vi "Test - Texture Mapping Test 1.vi"() -> ()   [LabVIEW 2020, in "3D.lvlib"]
uses:
  3D.lvlib
  Utility/Utility.lvlib
  Raster/Raster.lvlib
  Vector 3D.ctl
  Triangle 3D With Colour.ctl
  Raster/Rectangle Dimensions.ctl
  Camera.ctl
panel:
  in  "x Rotation":sgl(slide) scale=-180.0..180.0
  in  "y Rotation":sgl(slide) scale=0.0..360.0
  in  "z Rotation":sgl(slide) scale=-180.0..180.0
  in  "x Transform":sgl(slide) scale=-10.0..10.0
  in  "y Transform":sgl(slide)=5.0 scale=-10.0..10.0
  in  "z Transform":sgl(slide)=-18.0 scale=-20.0..10.0
  out "2D Picture":picture
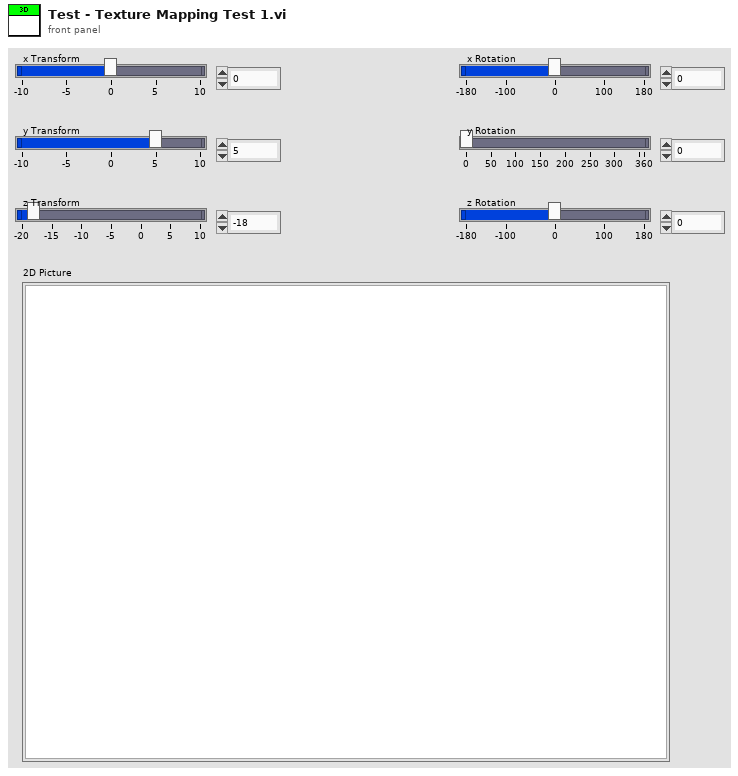
[diagram p1: front panel]
types:
  T1 = typedef "3D.lvlib/Vector 3D.ctl" = cluster{"x":sgl, "y":sgl, "z":sgl}
  T2 = typedef "3D.lvlib/Camera.ctl" = cluster{"Field Of View":sgl, "Near Plane":sgl, "Far Plane":sgl}
  T3 = typedef "Raster.lvlib/Rectangle Dimensions.ctl" = cluster{"Width":u32, "Height":u32}
  T4 = typedef "3D.lvlib/Object.ctl" = cluster{"Triangles":T5[], "Transform":T10, "Name":string, "Alpha Blending Enabled":bool, "Alpha":dbl, "Turntable Enabled":bool, "Material":T8}
  T5 = typedef "3D.lvlib/Triangle.ctl" = cluster{"Vertex 1":T6, "Vertex 2":T6, "Vertex 3":T6, "Alpha":dbl, "Alpha Blending Enabled":bool, "Colour":u32, "Material":T8}
  T6 = typedef "3D.lvlib/Vertex.ctl" = cluster{"Position":T1, "UV":T7, "Colour":u32}
  T7 = typedef "Raster.lvlib/UV.ctl" = cluster{"u":sgl, "v":sgl}
  T8 = typedef "3D.lvlib/Material.ctl" = cluster{"Diffuse Colour":u32, "Texture":T9}
  T9 = typedef "Raster.lvlib/Texture.ctl" = cluster{"Pixels":refnum<data-value>, "Size":T3}
  T10 = typedef "3D.lvlib/Transform.ctl" = cluster{"Position":T1, "Rotation":T1, "Scale":T1}
  T11 = typedef "3D.lvlib/Triangle 3D With Colour.ctl" = cluster{"Point 1":T1, "Point 2":T1, "Point 3":T1, "Fill Colour":u32, "Alpha":dbl, "Alpha Blending Enabled":bool, "Index":i32}
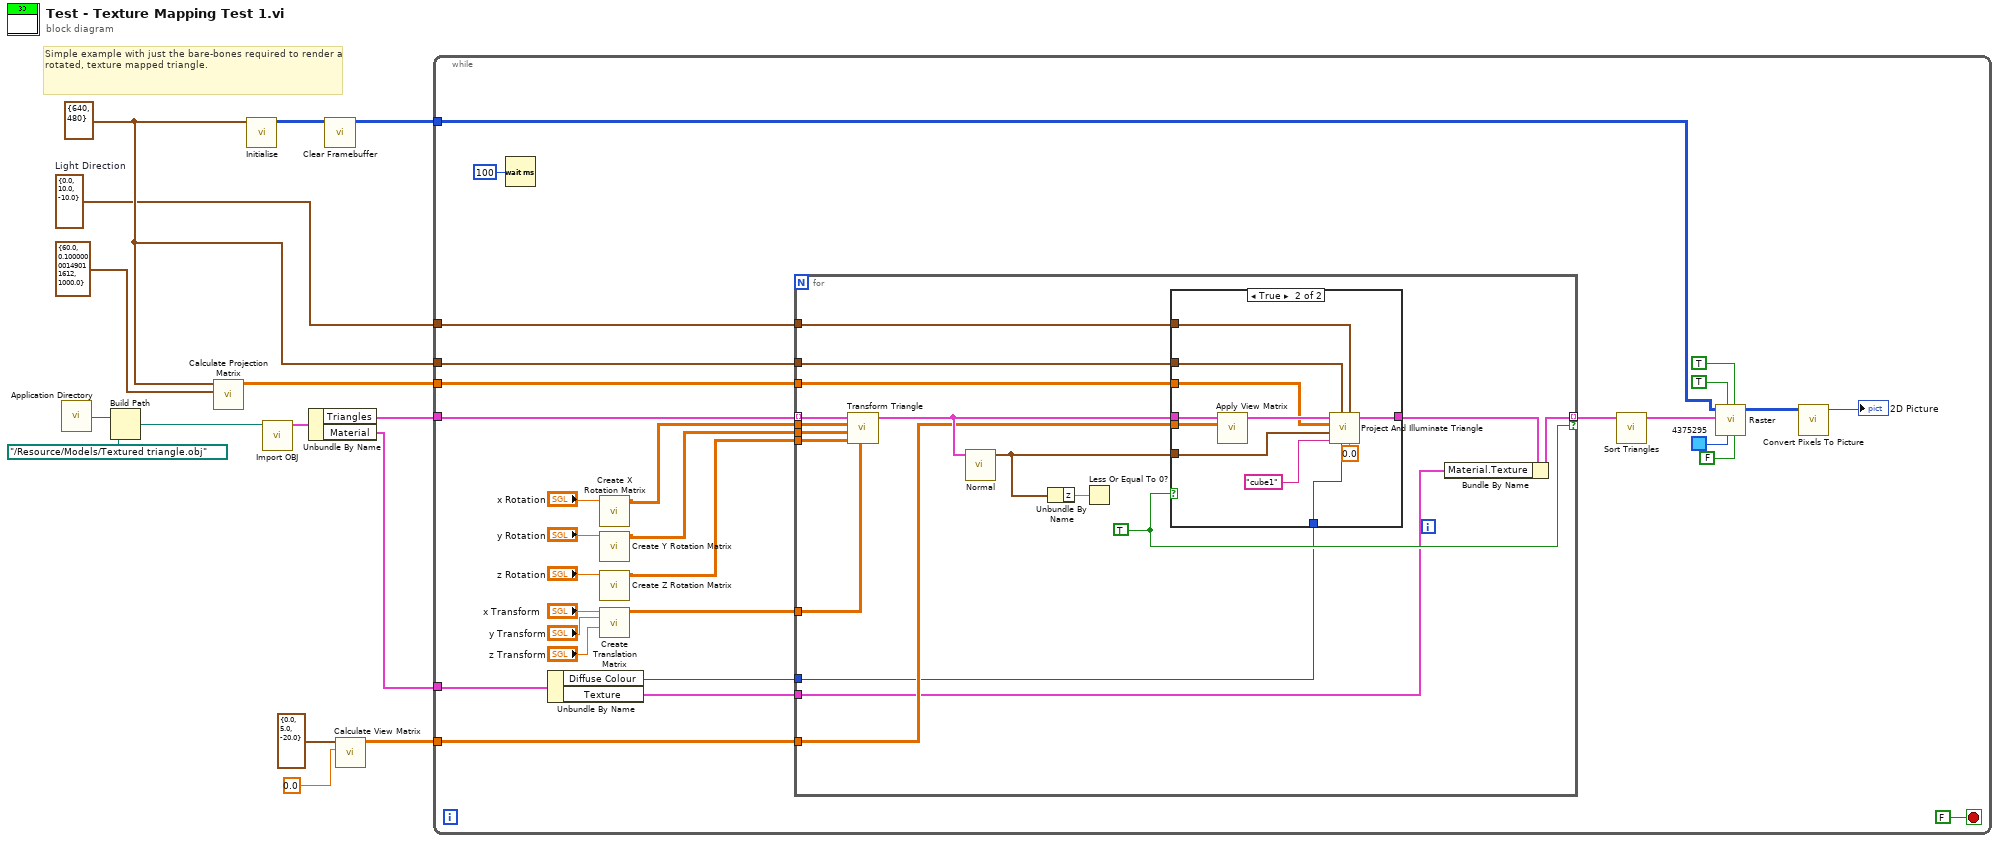
[diagram p0: block diagram]
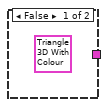
[diagram p2: hidden frame]
diagram:
  w10 = T1 {"x"=0.0, "y"=10.0, "z"=-10.0}  # Light Direction
  w11 = T3 {"Width"=640, "Height"=480} ("Screen Dimensions")
  # "Simple example with just the bare-bones required to render a rotated, texture mapped triangle."
  n1 = call <vilib>:"Application Directory.vi"() -> ("Application Directory"=w1:path)
  n2 = Build Path(base path=w1, name or relative path=path "../Resource/Models/Textured triangle.obj") -> (appended path=w7:path)
  n3 = call "Calculate Projection Matrix.vi"("Camera"=T2 {"Field Of View"=60.0, "Near Plane"=0.1, "Far Plane"=1000.0}, "Screen Dimensions"=w11) -> ("Projection Matrix"=w9:sgl[][])  [unwired: 9 in]
  n4 = call "Initialise.vi"("Screen Dimensions"=w11) -> ("Pixel Data out"=w12:u32[][])  [unwired: 10 in]
  n5 = call "Import OBJ.vi"("Object"=w7) -> ("Object"=w14:T4)  [unwired: 9 in, 1 out]
  n6 = Unbundle By Name(w14) -> ("Triangles"=w6:T5[], "Material"=w5:T8)
  n7 = call "Clear Framebuffer.vi"("Pixel Data in"=w12) -> ("Pixel Data out"=w15:u32[][])  [unwired: 10 in]
  n8 = call "Calculate View Matrix.vi"("Camera Rotation"=sgl 0.0, "Camera Position"=T1 {"x"=0.0, "y"=5.0, "z"=-20.0} ("output cluster")) -> ("View Matrix"=w2:sgl[][])  [unwired: 9 in]
  n9 = while {
    tunnel: w15 -> [w24]
    tunnel: w11 -> [w33]
    tunnel: w10 -> [w32]
    tunnel: w9 -> [w31]
    tunnel: w6 -> [w29]
    tunnel: w5 -> [w19]
    tunnel: w2 -> [w18]
    stop <- FALSE stop-if-true
    n10 = Wait (ms)(milliseconds to wait=u32 100) -> ()  [unwired: 1 out]
    n11 = Unbundle By Name(w19) -> ("Diffuse Colour"=w17:u32, "Texture"=w16:T9)
    n12 = call "Create X Rotation Matrix.vi"("Theta (°)"="x Rotation") -> ("Rotation X Matrix"=w38:sgl[][])  [unwired: 10 in]
    n13 = call "Create Y Rotation Matrix.vi"("Theta (°)"="y Rotation") -> ("Rotation Y Matrix"=w37:sgl[][])  [unwired: 10 in]
    n14 = call "Create Z Rotation Matrix.vi"("Theta (°)"="z Rotation") -> ("Rotation Z Matrix"=w36:sgl[][])  [unwired: 10 in]
    n15 = call "Create Translation Matrix.vi"("z"="z Transform", "y"="y Transform", "x"="x Transform") -> ("Translation Matrix"=w35:sgl[][])  [unwired: 8 in]
    n16 = for {
      tunnel: w36 -> [w58]
      tunnel: w38 -> [w60]
      tunnel: [w46] -> w34 mode=indexing if=w50
      tunnel: w37 -> [w59]
      tunnel: w35 -> [w57]
      tunnel: w29 -> [w51] mode=indexing
      tunnel: w33 -> [w55]
      tunnel: w31 -> [w54]
      tunnel: w32 -> [w53]
      tunnel: w18 -> [w49]
      tunnel: w17 -> [w48]
      tunnel: w16 -> [w45]
      w50 = TRUE
      n17 = call "Transform Triangle.vi"("Translation Matrix"=w57, "Rotation Z Matrix"=w58, "Rotation Y Matrix"=w59, "Rotation X Matrix"=w60, "Triangle in"=w51) -> ("Triangle out"=w56:T5)  [unwired: 6 in]
      n18 = call "Normal.vi"("Triangle"=w56) -> ("Normal"=w61:T1)  [unwired: 10 in]
      n19 = Unbundle By Name(w61) -> ("z"=w52:sgl)
      n20 = Less Or Equal To 0?(x=w52) -> ()  [unwired: 1 out]
      n21 = case shown="True" w50 {
        tunnel: [_ w66] -> w47
        tunnel: w61 -> [_ w72]
        tunnel: w56 -> [_ w70]
        tunnel: w55 -> [_ w69]
        tunnel: w54 -> [_ w68]
        tunnel: w53 -> [_ w67]
        tunnel: w49 -> [_ w65]
        tunnel: w48 -> [_ w62]
        frame False {
          (unwired) T11 {"Point 1"={"x"=0.0, "y"=0.0, "z"=0.0}, "Point 2"={"x"=0.0, "y"=0.0, "z"=0.0}, "Point 3"={"x"=0.0, "y"=0.0, "z"=0.0}, "Fill Colour"=12517256, "Alpha"=0.0, "Alpha Blending Enabled"=FALSE, "Index"=0} ("Triangle")
        }
        frame True {
          n22 = call "Apply View Matrix.vi"("View Matrix"=w65, "Triangle in"=w70) -> ("Triangle out"=w71:T5)  [unwired: 9 in]
          n23 = call "Project And Illuminate Triangle.vi"("Alpha"=0.0, "Light Direction"=w67, "Diffuse Colour"=w62, "Screen Dimensions"=w69, "Name"="cube1", "Normal"=w72, "Projection Matrix"=w68, "Triangle in"=w71) -> ("Triangle out"=w66:T5)  [unwired: 3 in]
        }
      }
      n24 = Bundle By Name(cluster=w47, "Material.Texture"=w45) -> (w46:T5)
    }
    n25 = call "Sort Triangles.vi"("Triangles"=w34) -> ("Triangles Sorted"=w26:T5[])  [unwired: 10 in]
    n26 = call "Raster.vi"("Draw Lines"=FALSE, "Draw Triangles"=TRUE, "Line Colour"=u32 4375295, "Textured"=TRUE, "Triangles Sorted"=w26, "Pixel Data in"=w24) -> ("Pixel Data out"=w25:u32[][])  [unwired: 5 in]
    n27 = call "Convert Pixels To Picture.vi"("Pixel Data in"=w25) -> ("2D Picture"=→"2D Picture":picture)  [unwired: 9 in, 1 out]
  }
